vi "Table, Set Cell Value.vi"(5 "cell value":string, 6 "error in":errorcluster, 7 "column (0)":i32, 8 "row (0)":i32, 9 "Tbl Refnum":refnum<vi>) -> (0 "error out":errorcluster, 1 "column+1":i32, 2 "row+1":i32, 3 "Tbl Refnum out":refnum<vi>)   [LabVIEW 2010]
doc: "This function sets a single table cell string value."
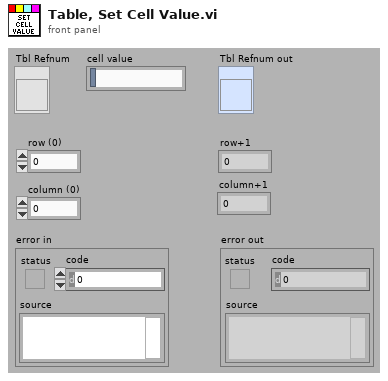
[diagram p1: front panel]
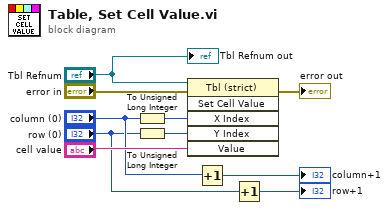
[diagram p0: block diagram]
diagram:
  n1 = To Unsigned Long Integer(number="column (0)") -> (unsigned 32bit integer=w2:u32)
  n2 = To Unsigned Long Integer(number="row (0)") -> (unsigned 32bit integer=w1:u32)
  n3 = invoke class="Tbl (strict)" method="Set Cell Value"(reference="Tbl Refnum", error in="error in", "X Index"=w2, "Y Index"=w1, "Value"="cell value") -> (error out=→"error out":errorcluster)  [unwired: 1 in, 5 out]
  n4 = Increment(x="column (0)") -> (x+1=→"column+1":i32)
  n5 = Increment(x="row (0)") -> (x+1=→"row+1":i32)
  "Tbl Refnum out" <- "Tbl Refnum"
